vi "beginPrepareRollToPassPlay.vi"(8 "error in (no error)":errorcluster, 9 "last command_interpreted":T1, 10 "Game":refnum<class "Game.lvclass">, 11 "PrepareRollToPassPlay in":refnum<class "PrepareRollToPassPlay.lvclass">) -> (0 "error out":errorcluster, 2 "BeginPrepareRollToPass?":bool, 3 "PrepareRollToPassPlay out":refnum<class "PrepareRollToPassPlay.lvclass">)   [LabVIEW 2023, in "PrepareRollToPassPlay.lvclass"]
uses:
  PrepareRollToPassPlay.lvclass
  Game_class/Game.lvclass
  Referee_class/command_interpreted.ctl
  Game_class/Game.lvclass/Game.ctl
  Referee_class/Referee.lvclass/Referee.ctl
  Parameters_class/Parameters.lvclass/Parameters.ctl
  Game_class/Read Referee.vi
  Game_class/Read Parameters.lvclass.vi
  Parameters_class/Read RollToPass.vi
  Referee_class/Read command_interpreted.vi
  Referee_class/Referee.lvclass
  Parameters_class/Parameters.lvclass
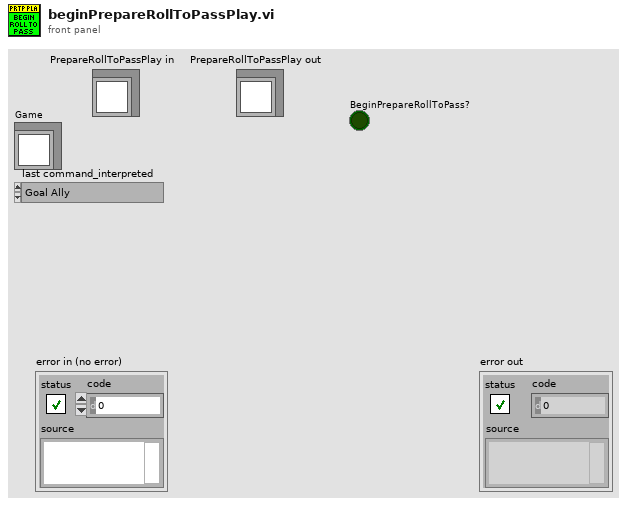
[diagram p1: front panel]
types:
  T1 = typedef "command_interpreted.ctl" = enum16{"Goal Ally", "Goal Enemy", "Ball Placement Enemy", "Ball Placement Ally", "Normal Half Time", "Extra Time  Break", "Extra Half Time", "None", "Post Game", "PKA Normal Start", "Prepare Kickoff Ally", "PKE Normal Start", "Prepare Kickoff Enemy", "Force Start", "Halt", "Timeout", "Prepare Penalty Ally", "Prepare Penalty Enemy", "PPA NormalStart", "PPE Normal Start", "Indirect Free Ally", "Direct Free Enemy", "Direct Free Ally", "Indirect Free Enemy", "Stop"}
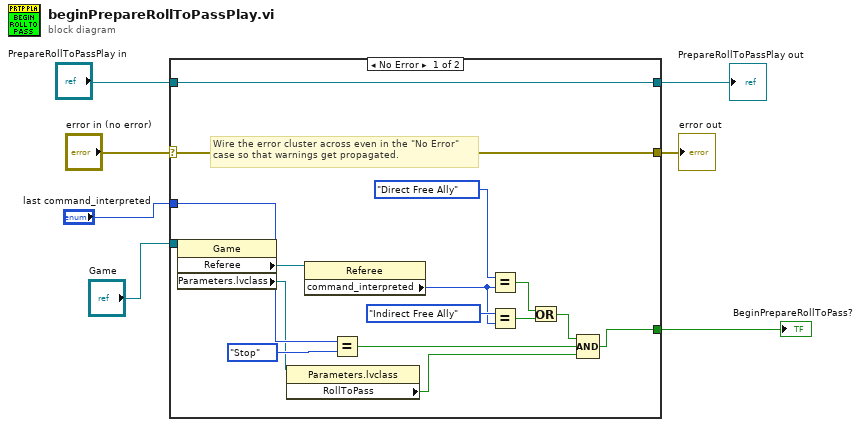
[diagram p0: block diagram]
diagram:
  n1 = case shown="No Error" "error in (no error)" {
    selector: "error in (no error)" -> [w22 w25]
    tunnel: [w22 w25] -> w6
    tunnel: [w23 w24] -> w1
    tunnel: "PrepareRollToPassPlay in" -> [w23 w24]
    tunnel: "Game" -> [w21 _]
    tunnel: [w12 _] -> w4
    tunnel: "last command_interpreted" -> [w10 _]
    frame No Error {
      # "Wire the error cluster across even in the \"No Error\"\ncase so that warnings get propagated."
      n2 = property class="Game"(reference=w21) -> ("Referee"=w20:refnum<class "Referee.lvclass">, "Parameters.lvclass"=w9:refnum<class "Parameters.lvclass">)  [unwired: 1 in, 2 out]
      n3 = property class="Parameters.lvclass"(reference=w9) -> ("RollToPass"=w8:bool)  [unwired: 1 in, 2 out]
      n4 = property class="Referee"(reference=w20) -> ("command_interpreted"=w16:T1)  [unwired: 1 in, 2 out]
      n5 = Equal?(x=w10, y=command_interpreted."Stop" ("command_interpreted")) -> (x = y?=w11:bool)
      n6 = Equal?(x=command_interpreted."Direct Free Ally" ("command_interpreted"), y=w16) -> (x = y?=w15:bool)
      n7 = Equal?(x=command_interpreted."Indirect Free Ally" ("command_interpreted"), y=w16) -> (x = y?=w13:bool)
      n8 = Or(x=w15, y=w13) -> (x .or. y?=w14:bool)
      n9 = Compound Arithmetic op=AND(w14, w11, w8) -> (w12:bool)
    }
    frame Error {
    }
  }
  "error out" <- w6
  "BeginPrepareRollToPass?" <- w4
  "PrepareRollToPassPlay out" <- w1
